vi "rt_loop_commands_receiving.vi"(11 "Message Queue":refnum<queue> caption="消息队列") -> ()   [LabVIEW 2015]
doc: "使用该模板构建简单状态机设计模式。各状态执行代码并决定转移状态。"
uses:
  support_vis/message_queue/message_cluster.ctl
  type_definitions/rt_loop_ui_communication_state.ctl
  globals/global_all_rt_loop_stop.vi
  globals/global_configuration_options.vi
  globals/global_rt_stream_connections.vi
  support_vis/message_queue/message_queue.lvlib
  <resource>/objmgr/ni.dex.rc
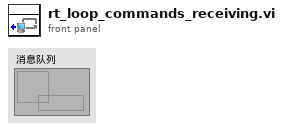
[diagram p1: front panel]
types:
  T1 = typedef "rt_loop_ui_communication_state.ctl" = enum16{"Initialize", "Listen for UI Writer", "Receive UI Commands"}
  T2 = typedef "message_queue.lvlib/message_cluster.ctl" = cluster{"Message":string, "Message Data":variant}
  T3 = typedef "Message Queue.lvlib/Message Cluster.ctl" = cluster{"Message":string, "Message Data":variant}
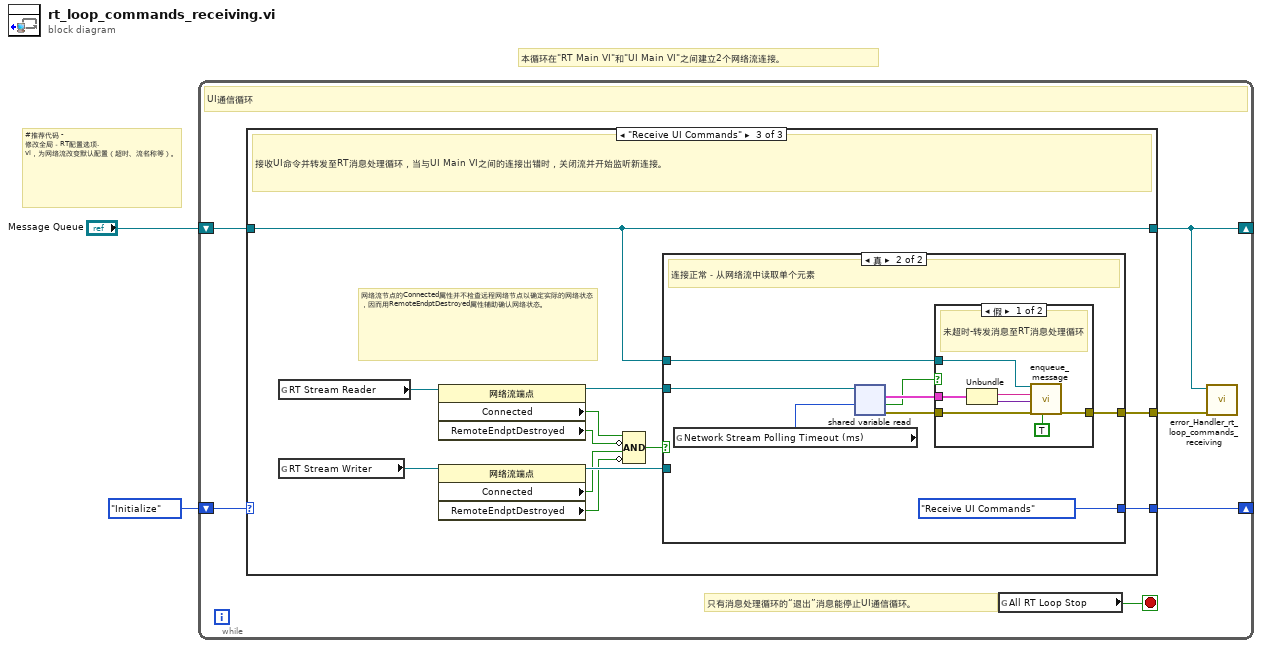
[diagram p0: block diagram]
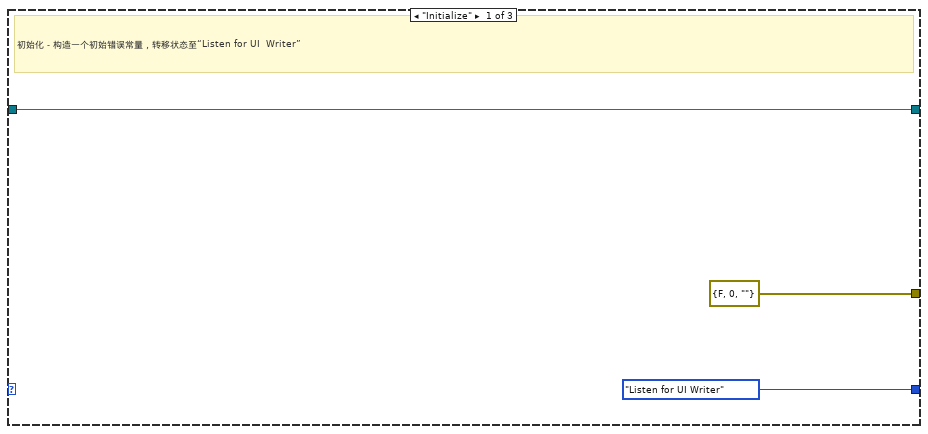
[diagram p2: hidden frame]
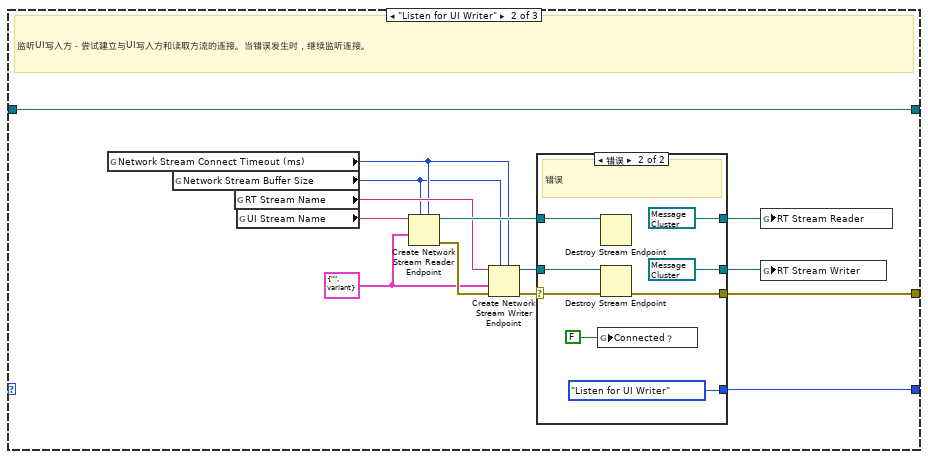
[diagram p3: hidden frame]
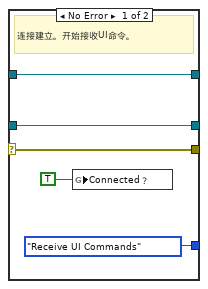
[diagram p4: hidden frame]
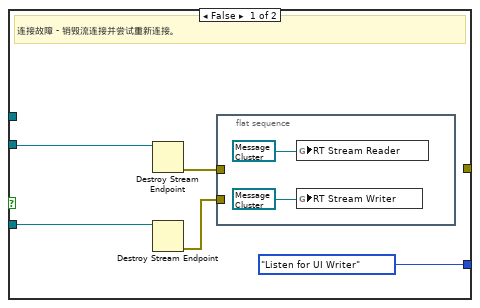
[diagram p5: hidden frame]
diagram:
  # "#推荐代码 -\n修改全局－RT配置选项.vi，为网络流改变默认配置（超时、流名称等）。"
  # "本循环在\"RT Main VI\"和\"UI Main VI\"之间建立2个网络流连接。"
  n1 = while {
    shift-right: [w7] -> _
    shift-left: rt_loop_ui_communication_state."Initialize" ("RT Loop - Host Communication State") -> [w8]
    shift-right: [w3] -> _
    shift-left: "Message Queue" -> [w4]
    stop <- w6 stop-if-true
    # "只有消息处理循环的“退出”消息能停止UI通信循环。"
    # "UI通信循环"
    n2 = case shown="\"Receive UI Commands\"" w8 {
      tunnel: [rt_loop_ui_communication_state."Listen for UI Writer" ("RT Loop - Host Communication State") w24 w49] -> w7
      tunnel: [errorcluster {"status"=FALSE, "code"=0, "source"=""} ("error IO") w18 w50] -> w5
      tunnel: [w9 w16 w47] -> w3
      tunnel: w4 -> [w9 w16 w47]
      frame "Initialize" {
        # "初始化－构造一个初始错误常量，转移状态至“Listen for UI  Writer”"
      }
      frame "Listen for UI Writer" {
        w17 = T2 {"Message"="", "Message Data"=variant} ("Message Cluster")
        # "监听UI写入方－尝试建立与UI写入方和读取方流的连接。当错误发生时，继续监听连接。"
        n3 = global read "global_configuration_options.vi" "Network Stream Connect Timeout (ms)"() -> (w14:i32)
        n4 = global read "global_configuration_options.vi" "Network Stream Buffer Size"() -> (w13:i32)
        n5 = global read "global_configuration_options.vi" "RT Stream Name"() -> (w15:string)
        n6 = global read "global_configuration_options.vi" "UI Stream Name"() -> (w12:string)
        n7 = Create Network Stream Reader Endpoint(5:w14, 7:w13, 9:w17, 11:w12) -> (0:w23:errorcluster, 3:w25:refnum<k21>)  [unwired: 3 in]
        n8 = Create Network Stream Writer Endpoint(5:w14, 7:w13, 8:w23, 9:w17, 11:w15) -> (0:w19:errorcluster, 3:w22:refnum<k21>)  [unwired: 2 in]
        n9 = case shown="错误" w19 {
          selector: w19 -> [w27 w33]
          tunnel: w25 -> [w29 w35]
          tunnel: [rt_loop_ui_communication_state."Receive UI Commands" ("RT Loop - Host Communication State") rt_loop_ui_communication_state."Listen for UI Writer" ("RT Loop - Host Communication State")] -> w24
          tunnel: w22 -> [w28 w34]
          tunnel: [w29 refnum<k21> refnum] -> w21
          tunnel: [w28 refnum<k21> refnum] -> w20
          tunnel: [w27 w32] -> w18
          frame No Error {
            # "连接建立。开始接收UI命令。"
            n10 = global write "global_rt_stream_connections.vi" "Connected？"(TRUE ("Connected？")) -> ()
          }
          frame Error {
            # "错误"
            n11 = global write "global_rt_stream_connections.vi" "Connected？"(FALSE ("Connected？")) -> ()
            n12 = Destroy Stream Endpoint(11:w35) -> ()  [unwired: 1 in, 1 out]
            n13 = Destroy Stream Endpoint(8:w33, 11:w34) -> (0:w32:errorcluster)
          }
        }
        n14 = global write "global_rt_stream_connections.vi" "RT Stream Reader"(w21) -> ()
        n15 = global write "global_rt_stream_connections.vi" "RT Stream Writer"(w20) -> ()
      }
      frame "Receive UI Commands" {
        # "网络流节点的Connected属性并不检查远程网络节点以确定实际的网络状态，因而用RemoteEndptDestroyed属性辅助确认网络状态。"
        # "接收UI命令并转发至RT消息处理循环，当与UI Main VI之间的连接出错时，关闭流并开始监听新连接。"
        n16 = global read "global_rt_stream_connections.vi" "RT Stream Reader"() -> (w45:refnum<k21>)
        n17 = global read "global_rt_stream_connections.vi" "RT Stream Writer"() -> (w48:refnum<k21>)
        n18 = property class="网络流端点"(reference=w45) -> (reference out=w43:refnum<k21>, "Connected"=w42:bool, "RemoteEndptDestroyed"=w41:bool)  [unwired: 1 in, 1 out]
        n19 = property class="网络流端点"(reference=w48) -> (reference out=w46:refnum<k21>, "Connected"=w40:bool, "RemoteEndptDestroyed"=w39:bool)  [unwired: 1 in, 1 out]
        n20 = Compound Arithmetic op=AND(w42, invert w41, w40, invert w39) -> (w44:bool)
        n21 = case shown="真" w44 {
          tunnel: [_ w65] -> w50
          tunnel: [rt_loop_ui_communication_state."Listen for UI Writer" ("RT Loop - Host Communication State") rt_loop_ui_communication_state."Receive UI Commands" ("RT Loop - Host Communication State")] -> w49
          tunnel: w47 -> [_ w64]
          tunnel: w46 -> [w52 _]
          tunnel: w43 -> [w51 w62]
          frame False {
            # "连接故障 - 销毁流连接并尝试重新连接。"
            n22 = Destroy Stream Endpoint(11:w51) -> (0:w53:errorcluster)  [unwired: 1 in]
            n23 = Destroy Stream Endpoint(11:w52) -> (0:w54:errorcluster)  [unwired: 1 in]
            n24 = flat-sequence {
              tunnel: w54 -> [_]
              tunnel: w53 -> [_]
              frame #0 {
                n25 = global write "global_rt_stream_connections.vi" "RT Stream Reader"(refnum<k21> refnum ("Host Writer Stream")) -> ()
                n26 = global write "global_rt_stream_connections.vi" "RT Stream Writer"(refnum<k21> refnum ("RT Writer Stream")) -> ()
              }
            }
          }
          frame True {
            # "连接正常－从网络流中读取单个元素"
            n27 = global read "global_configuration_options.vi" "Network Stream Polling Timeout (ms)"() -> (w58:i32)
            n28 = shared-variable-read(w62, w58) -> (w60:errorcluster, w59:bool, w61:T3)  [unwired: 1 in, 1 out]
            n29 = case shown="假" w59 {
              tunnel: [w69 w73] -> w65
              tunnel: w64 -> [w70 _]
              tunnel: w61 -> [w68 _]
              tunnel: w60 -> [w67 w73]
              frame False {
                # "未超时-转发消息至RT消息处理循环"
                n30 = Unbundle(w68) -> ("Message"=w72:string, "Message Data"=w71:variant)
                n31 = call "enqueue_message.vi"("Priority Message? (F)"=TRUE, "error in (no error)"=w67, "Message Data"=w71, "Message"=w72, "Message Queue"=w70) -> ("error out"=w69:errorcluster)  [unwired: 5 in, 1 out]
              }
              frame True {
                # "超时－无新命令"
              }
            }
          }
        }
      }
    }
    n32 = global read "global_all_rt_loop_stop.vi" "All RT Loop Stop"() -> (w6:bool)
    n33 = call "error_Handler_rt_loop_commands_receiving.vi"("error in (no error)"=w5, "Message Queue"=w3) -> ()  [unwired: 9 in, 1 out]
  }
